vi "SLSC Export Configuration.vi"(0 "path":path, 1 "Loop rate":u32, 2 "Description":string, 5 "SLSC EDS module in":T2, 7 "Custom Device Name":string, 9 "Channels to Enable":string[](array[string]), 11 "error in (no error)":errorcluster, 12 "Apply Default":bool, 14 "Apply Reset":bool) -> (15 "error out":errorcluster)   [LabVIEW 2019, in "SLSC EDS System Explorer.lvlib"]
uses:
  SLSC EDS System Explorer.lvlib
  SLSC EDS API/JSON parsing/EDSjsonStructure.ctl
  SLSC EDS API/JSON parsing/enum.ctl
  SLSC EDS API/JSON parsing/property.ctl
  SLSC EDS API/JSON parsing/command.ctl
  SLSC EDS API/JSON parsing/scale.ctl
  SLSC EDS API/JSON parsing/physicalChannel.ctl
  SLSC EDS API/JSON parsing/register.ctl
  SLSC EDS API/JSON parsing/EDS_Custom_Device_Structure.ctl
  <vilib>/addons/_JKI.lib/Serialization/JSON/JKI JSON Serialization.lvlib
panel:
  in  "Value":T1
  # "not working\nregisterMap->registers->initialValue"
  # "not working\nregisterMap->registers->initialValue"
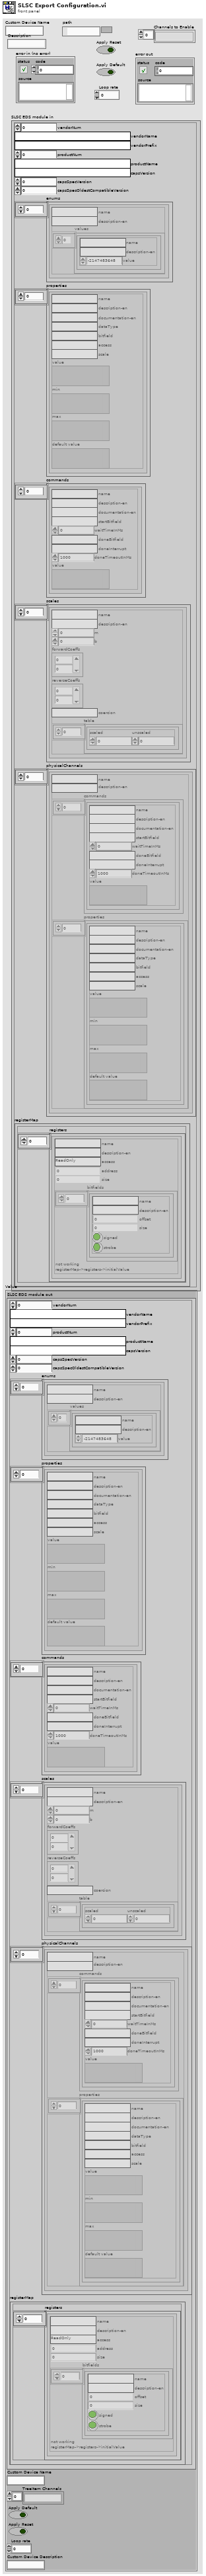
[diagram p1: front panel]
types:
  T1 = typedef "EDS_Custom_Device_Structure.ctl" = cluster{"SLSC EDS module out":T2, "Custom Device Name":string, "TreeItem Channels":string[], "Apply Default":bool, "Apply Reset":bool, "Loop rate":u32, "Custom Device Description":string}
  T2 = typedef "EDSjsonStructure.ctl" = cluster{"vendorNum":u32, "vendorName":string, "vendorPrefix":string, "productNum":u32, "productName":string, "capsVersion":string, "capsSpecVersion":u32, "capsSpecOldestCompatibleVersion":u32, "enums":T3[], "properties":T4[], "commands":T5[], "scales":T6[], "physicalChannels":T7[], "registerMap":cluster{"registers":T8[]}}
  T3 = typedef "enum.ctl" = cluster{"name":string, "description-en":string, "values":cluster{"name":string, "description-en":string, "value":i32}[]}
  T4 = typedef "property.ctl" = cluster{"name":string, "description-en":string, "documentation-en":string, "dataType":string, "bitfield":string, "access":string, "scale":string, "value":variant, "min":variant, "max":variant, "default value":variant}
  T5 = typedef "command.ctl" = cluster{"name":string, "description-en":string, "documentation-en":string, "startBitfield":string, "waitTimeInMs":i32, "doneBitfield":string, "doneInterrupt":string, "doneTimeoutInMs":i32, "value":variant}
  T6 = typedef "scale.ctl" = cluster{"name":string, "description-en":string, "m":dbl, "b":dbl, "forwardCoeffs":dbl[], "reverseCoeffs":dbl[], "coercion":string, "table":cluster{"scaled":dbl, "unscaled":dbl}[]}
  T7 = typedef "physicalChannel.ctl" = cluster{"name":string, "description-en":string, "commands":T5[], "properties":T4[]}
  T8 = typedef "register.ctl" = cluster{"name":string, "description-en":string, "access":string, "address":u32, "size":u32, "bitfields":cluster{"name":string, "description-en":string, "offset":u32, "size":u32, "signed":bool, "strobe":bool}[]}
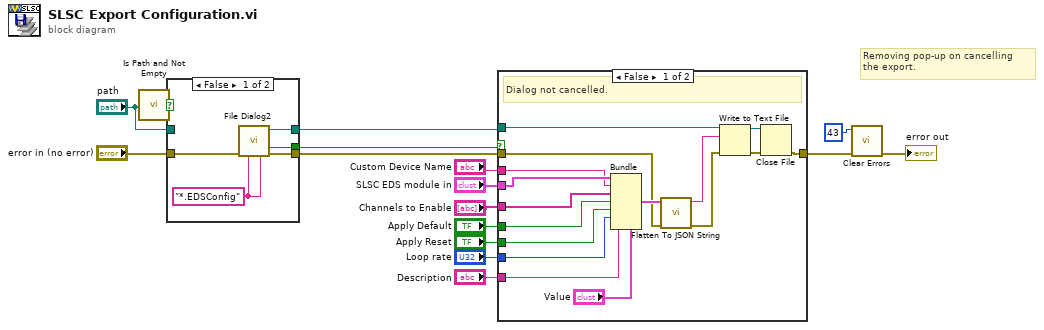
[diagram p0: block diagram]
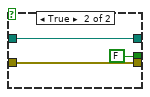
[diagram p2: hidden frame]
diagram:
  # "Removing pop-up on cancelling\nthe export."
  n1 = call <vilib>:"Is Path and Not Empty.vi"("path"="path") -> ("Is Path and Not Empty?"=w9:bool)  [unwired: 4 in]
  n2 = case shown="False" w9 {
    tunnel: [w21 FALSE ("cancelled")] -> w5
    tunnel: "error in (no error)" -> [w20 w23]
    tunnel: [w19 w23] -> w6
    tunnel: [w18 w24] -> w4
    tunnel: "path" -> [_ w24]
    frame False {
      w17 = "*.EDSConfig" ("pattern label")
      n3 = call "File Dialog2"("error in"=w20, "pattern (all files)"=w17, "pattern label"=w17) -> ("selected path"=w18:path, "cancelled"=w21:bool, "error out"=w19:errorcluster)  [unwired: 9 in, 1 out]
    }
    frame True {
    }
  }
  n4 = case shown="False" w5 {
    tunnel: w4 -> [w39 _]
    tunnel: "SLSC EDS module in" -> [w26 _]
    tunnel: [w33 w41] -> w11
    tunnel: w6 -> [w30 w41]
    tunnel: "Apply Reset" -> [w31 _]
    tunnel: "Apply Default" -> [w32 _]
    tunnel: "Loop rate" -> [w36 _]
    tunnel: "Channels to Enable" -> [w29 _]
    tunnel: "Custom Device Name" -> [w25 _]
    tunnel: "Description" -> [w28 _]
    frame False {
      # "Dialog not cancelled."
      n5 = Bundle(cluster="Value", "SLSC EDS module out"=w26, "Custom Device Name"=w25, "TreeItem Channels"=w29, "Apply Default"=w32, "Apply Reset"=w31, "Loop rate"=w36, "Custom Device Description"=w28) -> (w38:T1)
      n6 = call <vilib>:"Flatten To JSON String.vi"("error in (no error)"=w30, "Variant"=w38) -> ("error out"=w37:errorcluster, "JSON String"=w40:string)  [unwired: 8 in]
      n7 = Write to Text File(file (use dialog)=w39, text=w40, error in=w37) -> (refnum out=w35:refnum<file>, error out=w34:errorcluster)  [unwired: 1 in, 1 out]
      n8 = Close File(refnum=w35, error in=w34) -> (error out=w33:errorcluster)  [unwired: 1 out]
    }
    frame True {
      # "The dialog was cancelled."
    }
  }
  n9 = call <vilib>:"Clear Errors.vi"("error in (no error)"=w11, "specific error code to clear (0: all)"=43) -> ("error out"=→"error out":errorcluster)  [unwired: 4 in, 1 out]
